vi "SW_Load_data_for_Analysis_from_TDMS.vi"(4 "Data samples to load":i64=-1, 6 "create index file? (T)":bool, 8 "error in (no error)":errorcluster, 9 "Progress bar reference":refnum<vi>, 10 "Cluster of paths input":T3, 11 "Data flow controls":T4) -> (0 "error out":errorcluster, 2 "Time to load, ms":u32, 3 "Loaded data":T1={"Absolute timestamp (DBL)"=[], "Relative timestamp (DBL)"=[], "Zones normalized allocation array"=[], "Coordinates and speed"=[], "Current zone and TTLs"=[], "Acquisition settings cluster out"={"Researcher name"="", "N segments MIDFIELD"=0, "N segments BORDER"=0, "Radius, mm CENTER"=0, "Radius, mm MIDFIELD"=0, "Starting angle MIDFIELD"=0, "Starting angle BORDER"=0, "Cage diameter, mm"=0, "Bridge swap"=FALSE, "Bridge V. offset"=0.0, "Twisted neck"=FALSE, "Offset H."=0.0, "Name prefix"="SavedTrack", "Stop at"=0.0, "\"Stop at\" enabled"=FALSE, "Settings loaded OK"=FALSE}, "Stimulus presets array"=[]} {"Acquisition settings cluster out"."Stop at" format="%<%H:%M:%S>t"}, 5 "Data loaded OK":bool, 7 "Settings loaded OK":bool)   [LabVIEW 2018, in "Tracker.lvlib"]
uses:
  Tracker.lvlib
panel:
  out "Author's name":string
  out "Stimulus presets array (loaded)":T2(array[cluster])
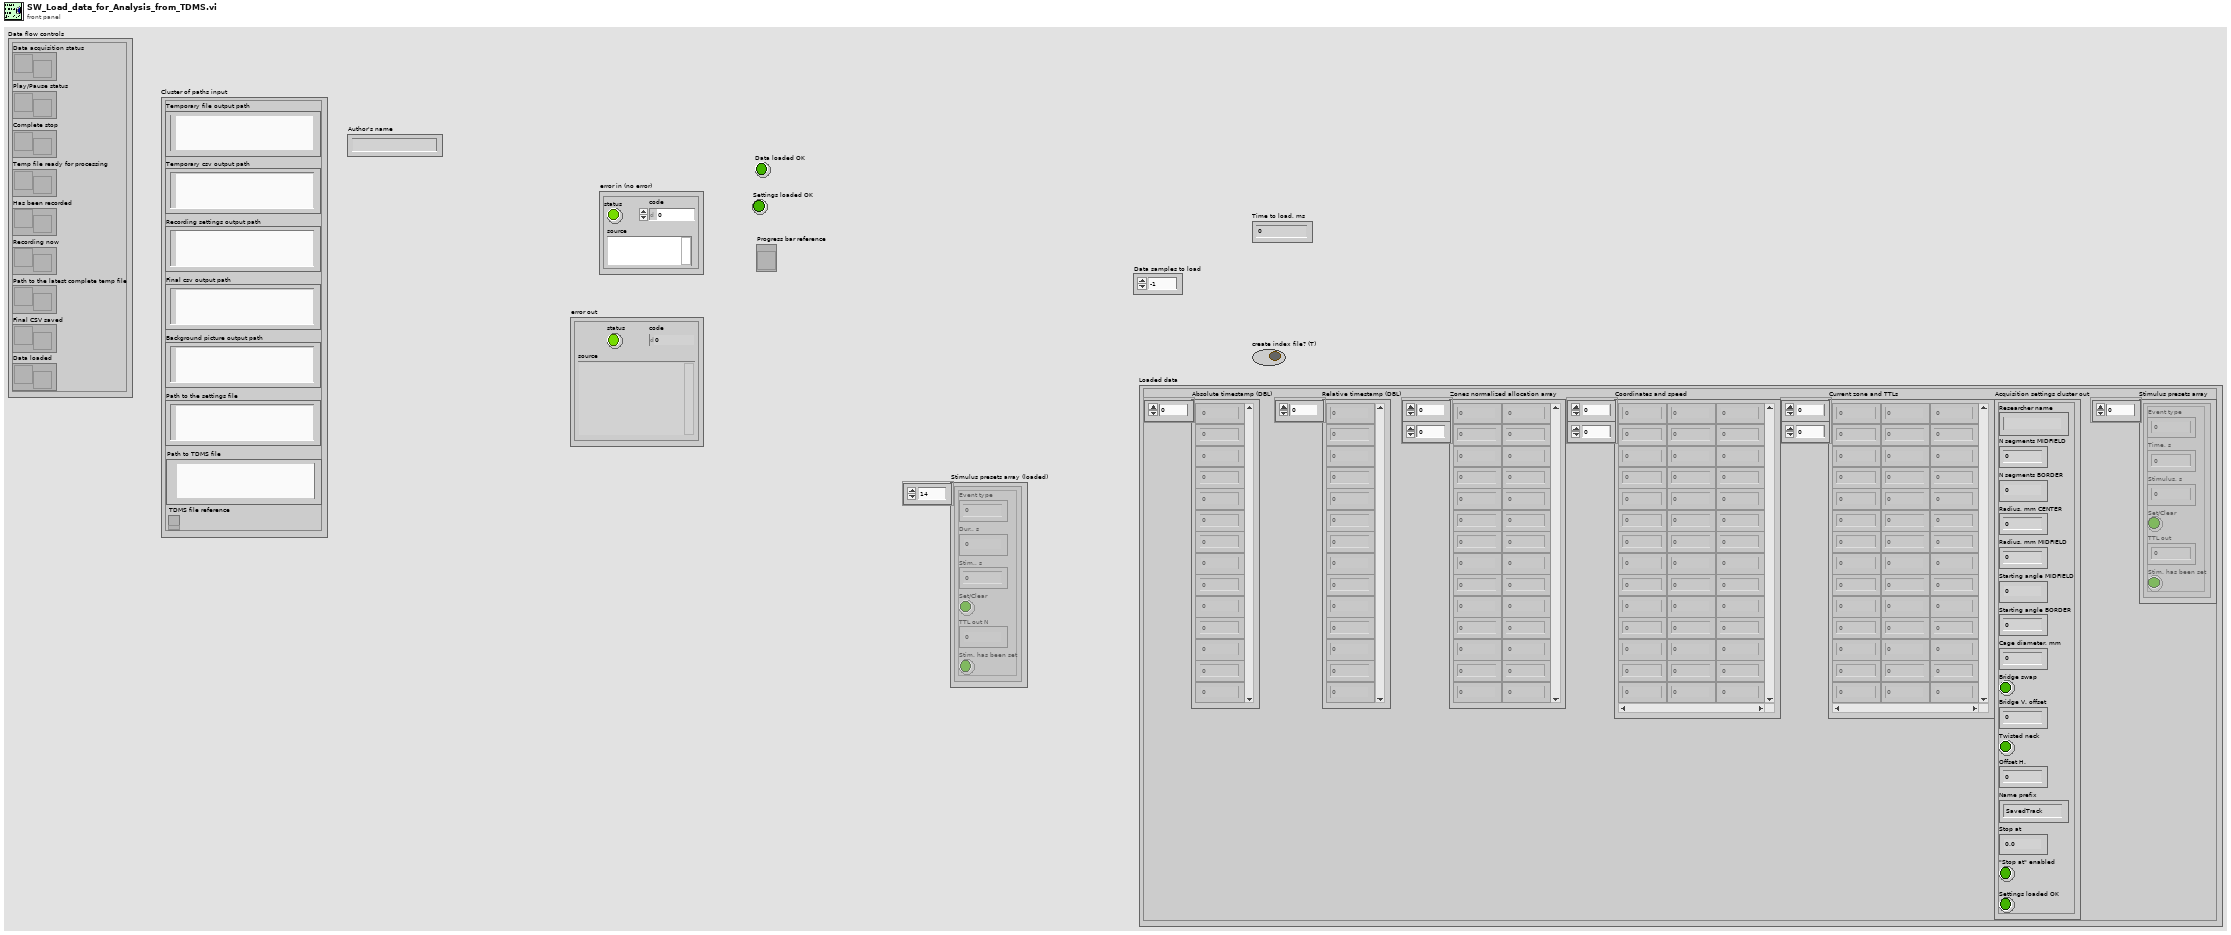
[diagram p1: front panel]
types:
  T1 = cluster{"Absolute timestamp (DBL)":dbl[], "Relative timestamp (DBL)":dbl[], "Zones normalized allocation array":dbl[][], "Coordinates and speed":dbl[][], "Current zone and TTLs":u8[][], "Acquisition settings cluster out":cluster{"Researcher name":string, "N segments MIDFIELD":u8, "N segments BORDER":u8, "Radius, mm CENTER":u16, "Radius, mm MIDFIELD":u16, "Starting angle MIDFIELD":i16, "Starting angle BORDER":i16, "Cage diameter, mm":u16, "Bridge swap":bool, "Bridge V. offset":sgl, "Twisted neck":bool, "Offset H.":sgl, "Name prefix":string, "Stop at":dbl, "\"Stop at\" enabled":bool, "Settings loaded OK":bool}, "Stimulus presets array":cluster{"Event type":u16, "Time, s":sgl, "Stimulus, s":sgl, "Set/Clear":bool, "TTL out":u16, "Stim. has been set":bool}[]}
  T2 = cluster{"Event type":u16, "Dur., s":sgl, "Stim., s":sgl, "Set/Clear":bool, "TTL out N":u16, "Stim. has been set":bool}[]
  T3 = cluster{"Temporary file output path":path, "Temporary csv output path":path, "Recording settings output path":path, "Final csv output path":path, "Background picture output path":path, "Path to the settings file":path, "Path to TDMS file":path, "TDMS file reference":refnum<k34>}
  T4 = cluster{"Data acquisition status":refnum<notifier>, "Play/Pause status":refnum<notifier>, "Complete stop":refnum<notifier>, "Temp file ready for processing":refnum<notifier>, "Has been recorded":refnum<notifier>, "Recording now":refnum<notifier>, "Path to the latest complete temp file":refnum<notifier>, "Final CSV saved":refnum<notifier>, "Data loaded":refnum<notifier>}
  T5 = cluster{"N segments BORDER":u8, "Starting angle BORDER":i16, "N segments MIDFIELD":u8, "Starting angle MIDFIELD":i16, "Radius, mm MIDFIELD":u16, "Amount of central segments":u8, "Radius, mm CENTER":u16, "Bridge swap":bool, "Bridge V. offset":sgl, "Twisted neck":bool, "Offset H.":sgl, "Zones configuration":string[], "IO parameters string":string, "Cage diameter, mm":u16, "Name prefix":string, "Stop at":dbl, "\"Stop at\" enabled":bool}
  T6 = enum16{"big-endian, network order", "native, host order", "little-endian"}
  T7 = enum16{"open", "open or create", "create or replace", "create", "open (read-only)"}
  T8 = cluster{"N segments BORDER":u8, "Starting angle BORDER":i16, "N segments MIDFIELD":u8, "Starting angle MIDFIELD":i16, "Radius, mm MIDFIELD":u16, "Amount of central segments":u8, "Radius, mm CENTER":u16, "Bridge offset":sgl, "Bridge swap":bool, "Zones configuration":string[], "IO parameters string":string, "Cage diameter, mm":u16}
  T9 = cluster{"Event type":u16, "Time, s":sgl, "Stimulus, s":sgl, "Set/Clear":bool, "TTL out":u16, "Stim. has been set":bool}
  T10 = cluster{string, "N segments MIDFIELD":u8, "N segments BORDER":u8, "Radius, mm CENTER":u16, "Radius, mm MIDFIELD":u16, "Starting angle MIDFIELD":i16, "Starting angle BORDER":i16, "Cage diameter, mm":u16, "Bridge swap":bool, "Bridge V. offset":sgl, "Twisted neck":bool, "Offset H.":sgl, "Name prefix":string, "Stop at":dbl, "\"Stop at\" enabled":bool, bool}
  T11 = cluster{dbl[], dbl[], "Zones normalized allocation array":dbl[][], dbl[][], u8[][], cluster{string, "N segments MIDFIELD":u8, "N segments BORDER":u8, "Radius, mm CENTER":u16, "Radius, mm MIDFIELD":u16, "Starting angle MIDFIELD":i16, "Starting angle BORDER":i16, "Cage diameter, mm":u16, "Bridge swap":bool, "Bridge V. offset":sgl, "Twisted neck":bool, "Offset H.":sgl, "Name prefix":string, "Stop at":dbl, "\"Stop at\" enabled":bool, bool}, cluster{"Event type":u16, "Time, s":sgl, "Stimulus, s":sgl, "Set/Clear":bool, "TTL out":u16, "Stim. has been set":bool}[]}
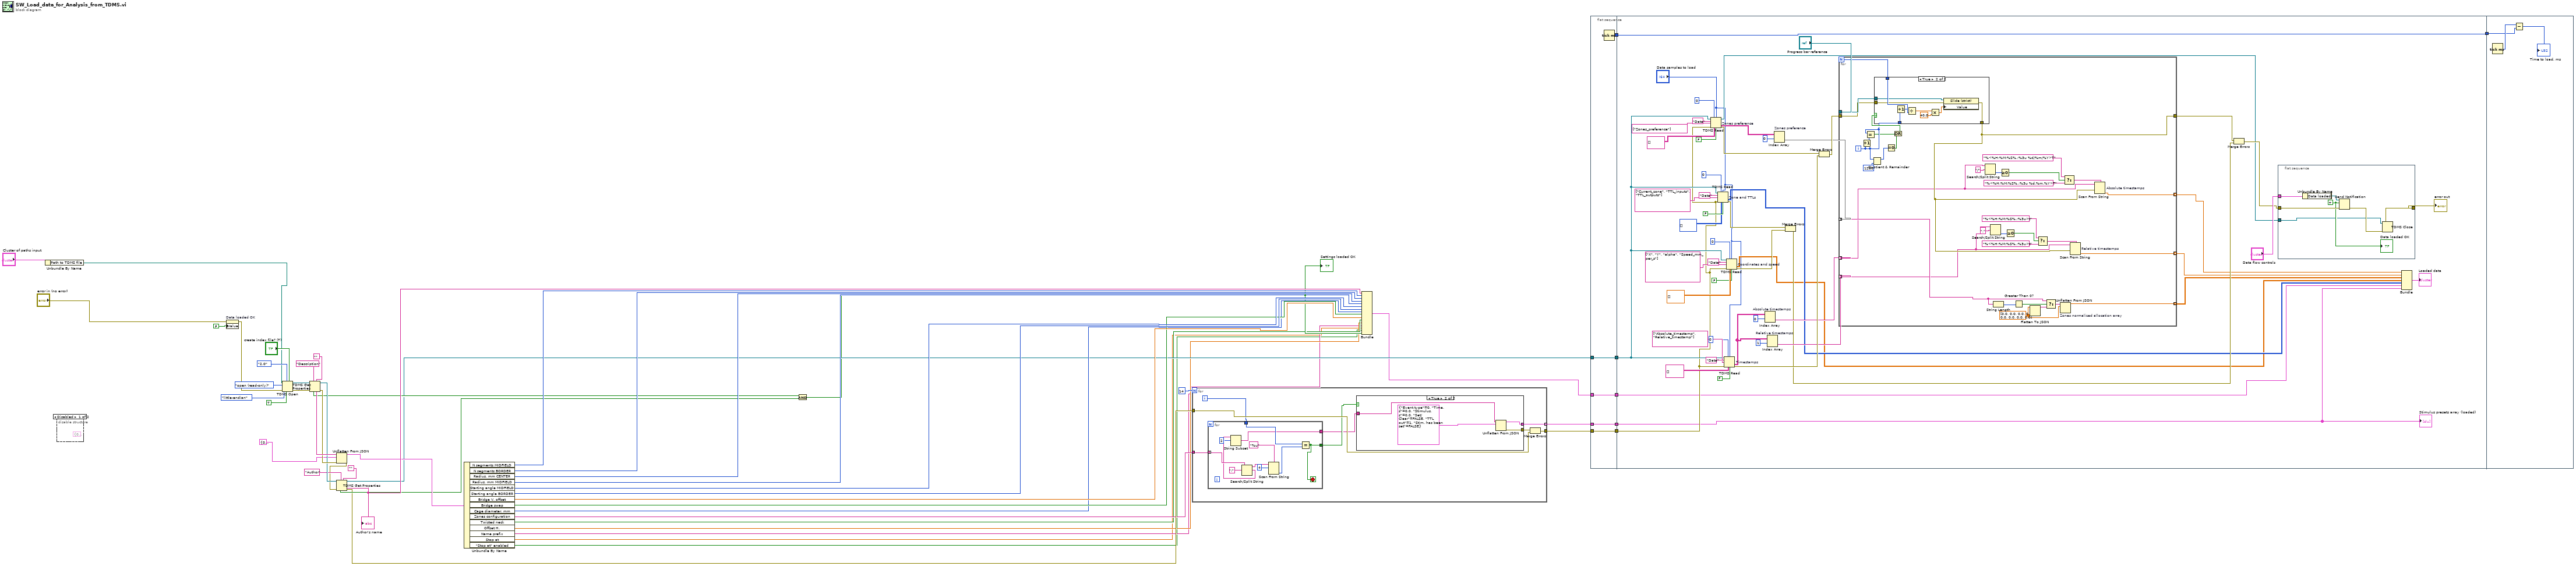
[diagram p0: block diagram]
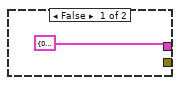
[diagram p4: hidden frame]
diagram:
  n1 = Unbundle By Name("Cluster of paths input") -> ("Path to TDMS file"=w9:path)
  n2 = disable-structure shown="Disabled" {
    frame Disabled {
      (unwired) T8 {"N segments BORDER"=0, "Starting angle BORDER"=0, "N segments MIDFIELD"=0, "Starting angle MIDFIELD"=0, "Radius, mm MIDFIELD"=0, "Amount of central segments"=0, "Radius, mm CENTER"=0, "Bridge offset"=0.0, "Bridge swap"=FALSE, "Zones configuration"=[], "IO parameters string"="[12,1,1,0,0,0]", "Cage diameter, mm"=180} ("Parameters")
    }
    frame Enabled {
    }
  }
  n3 = property on="Data loaded OK" class="Bool (strict)"(error in="error in (no error)", "Value"=FALSE ("Data loaded OK")) -> (error out=w17:errorcluster)  [unwired: 1 in, 1 out]
  n4 = TDMS Open(5:"create index file? (T)", 6:TRUE ("disable buffering? (T)"), 7:enum16{"1.0", "2.0"}."2.0" ("file format version (2.0)"), 8:w17, 9:T6."little-endian" ("byte order (2:little-endian)"), 10:T7."open (read-only)" ("operation (0:open)"), 11:w9) -> (0:w46:errorcluster, 3:w47:refnum<k34>)
  n5 = TDMS Get Properties(5:"", 7:"Description" ("property name"), 8:w46, 11:w47) -> (0:w42:errorcluster, 3:w41:refnum<k34>, 4:w43:string, 6:w26:bool)  [unwired: 2 in, 2 out]
  n6 = Unflatten From JSON(JSON string=w43, type and defaults=T5 {"N segments BORDER"=0, "Starting angle BORDER"=0, "N segments MIDFIELD"=0, "Starting angle MIDFIELD"=0, "Radius, mm MIDFIELD"=0, "Amount of central segments"=0, "Radius, mm CENTER"=0, "Bridge swap"=FALSE, "Bridge V. offset"=0.0, "Twisted neck"=FALSE, "Offset H."=0.0, "Zones configuration"=[], "IO parameters string"="[12,1,1,0,0,0]", "Cage diameter, mm"=180, "Name prefix"="SavedTrack", "Stop at"=0.0, "\"Stop at\" enabled"=FALSE} ("Parameters"), error in (no error)=w42) -> (value=w28:T5, error out=w38:errorcluster)  [unwired: 4 in]
  n7 = TDMS Get Properties(5:"", 7:"Author" ("property name"), 8:w38, 11:w41) -> (0:w24:errorcluster, 3:w21:refnum<k34>, 4:w37:string, 6:w25:bool)  [unwired: 2 in, 2 out]
  "Author's name" <- w37
  n8 = Unbundle By Name(w28) -> ("N segments MIDFIELD"=w36:u8, "N segments BORDER"=w35:u8, "Radius, mm CENTER"=w34:u16, "Radius, mm MIDFIELD"=w33:u16, "Starting angle MIDFIELD"=w32:i16, "Starting angle BORDER"=w31:i16, "Bridge V. offset"=w30:sgl, "Bridge swap"=w29:bool, "Cage diameter, mm"=w27:u16, "Zones configuration"=w23:string[], "Twisted neck"=w5:bool, "Offset H."=w4:sgl, "Name prefix"=w3:string, "Stop at"=w2:dbl, "\"Stop at\" enabled"=w1:bool)
  n9 = And(x=w26, y=w25) -> (x .and. y?=w6:bool)
  "Settings loaded OK" <- w6
  n10 = for {
    N: 14 -> [_]
    tunnel: w24 -> [w58]
    tunnel: [w60] -> w20
    tunnel: [w61] -> w19 mode=indexing
    tunnel: w23 -> [w56]
    i -> [w57]
    n11 = for {
      tunnel: w56 -> [w72] mode=indexing
      tunnel: w57 -> [w66]
      tunnel: [w65] -> w55
      tunnel: [w64] -> w54
      stop <- w65 stop-if-true
      n12 = Search/Split String(string=w72, search string/char (-)=":") -> (substring before match=w70:string, match + rest of string=w63:string)  [unwired: 1 in, 1 out]
      n13 = String Subset(string=w63, offset (0)=2) -> (substring=w64:string)  [unwired: 1 in]
      n14 = Scan From String(format string="%u", input string=w70, initial scan location=u32 4) -> (output 1=w67:u32)  [unwired: 2 in, 3 out]
      n15 = Equal?(x=w66, y=w67) -> (x = y?=w65:bool)
    }
    n16 = case shown="True" w55 {
      tunnel: w54 -> [_ w77]
      tunnel: [T9 {"Event type"=0, "Time, s"=0.0, "Stimulus, s"=0.0, "Set/Clear"=FALSE, "TTL out"=1, "Stim. has been set"=FALSE} ("Cluster of the stimuls settings") w76] -> w61
      tunnel: [_ w75] -> w59
      frame False {
      }
      frame True {
        n17 = Unflatten From JSON(JSON string=w77, type and defaults=T9 {"Event type"=0, "Time, s"=0.0, "Stimulus, s"=0.0, "Set/Clear"=FALSE, "TTL out"=1, "Stim. has been set"=FALSE} ("Cluster of the stimuls settings")) -> (value=w76:T9, error out=w75:errorcluster)  [unwired: 5 in]
      }
    }
    n18 = Merge Errors(w59, w58) -> (w60:errorcluster)
  }
  n19 = Bundle(w37, "N segments MIDFIELD"=w36, "N segments BORDER"=w35, "Radius, mm CENTER"=w34, "Radius, mm MIDFIELD"=w33, "Starting angle MIDFIELD"=w32, "Starting angle BORDER"=w31, "Cage diameter, mm"=w27, "Bridge swap"=w29, "Bridge V. offset"=w30, "Twisted neck"=w5, "Offset H."=w4, "Name prefix"=w3, "Stop at"=w2, "\"Stop at\" enabled"=w1, w6) -> (w8:T10)  [unwired: 1 in]
  n20 = flat-sequence {
    tunnel: w19 -> [w79]
    tunnel: w8 -> [w80]
    tunnel: w20 -> [w81]
    tunnel: w21 -> [w82]
    tunnel: [w82] -> w15
    tunnel: [w81] -> w14
    tunnel: [w80] -> w13
    tunnel: [w79] -> w12
    tunnel: [w78] -> w11
    tunnel: w15 -> [w117]
    tunnel: w14 -> [w116]
    tunnel: w13 -> [w83]
    tunnel: w12 -> [w95]
    tunnel: w11 -> [w84]
    tunnel: [w84] -> w10
    tunnel: w10 -> [w187]
    frame #0 {
      n21 = Tick Count (ms)() -> (millisecond timer value=w78:u32)
    }
    frame #1 {
      n22 = TDMS Read "Zones preference"(0:w117, 1:i64 0 ("offset (0)"), 2:"Data samples to load", 5:"Data" ("group name in"), 7:string[] ["Zones_preference"] ("Columns Names"), 11:w116, 12:string[][] [], 13:FALSE ("return channels in file order? (F)")) -> (4:w90:refnum<k34>, 10:w102:string[][], 15:w113:errorcluster)  [unwired: 3 out]
      n23 = TDMS Read "Zone and TTLs"(0:w117, 1:i64 0 ("offset (0)"), 2:"Data samples to load", 5:"Data" ("group name in"), 7:string[] ["Current_zone", "TTL_inputs", "TTL_outputs"] ("Columns Names"), 11:w116, 12:u8[][] [], 13:FALSE ("return channels in file order? (F)")) -> (10:w93:u8[][], 15:w111:errorcluster)  [unwired: 4 out]
      n24 = TDMS Read "Timestamps"(0:w117, 1:i64 0 ("offset (0)"), 2:"Data samples to load", 5:"Data" ("group name in"), 7:string[] ["Absolute_timestamp", "Relative_timestamp"] ("Columns Names"), 11:w116, 12:string[][] [], 13:FALSE ("return channels in file order? (F)")) -> (10:w106:string[][], 15:w112:errorcluster)  [unwired: 4 out]
      n25 = TDMS Read "Coordinates and speed"(0:w117, 1:i64 0 ("offset (0)"), 2:"Data samples to load", 5:"Data" ("group name in"), 7:string[] ["X", "Y", "alpha", "Speed_mm_per_s"] ("Columns Names"), 11:w116, 12:dbl[][] [], 13:FALSE ("return channels in file order? (F)")) -> (10:w92:dbl[][], 15:w100:errorcluster)  [unwired: 4 out]
      n26 = Index Array "Absolute timestamps"(array=w106, index (row)=0) -> (element=w105:string[])  [unwired: 1 in]
      n27 = Index Array "Relative timestamps"(array=w106, index (row)=1) -> (element=w104:string[])  [unwired: 1 in]
      n28 = Index Array "Zones preference"(array=w102, index (row)=0) -> (element=w101:string[])  [unwired: 1 in]
      n29 = Merge Errors(w111, w100) -> (w99:errorcluster)
      n30 = Merge Errors(w113, w112) -> (w114:errorcluster)
      n31 = for {
        N -> [w168]
        tunnel: w114 -> [w166]
        tunnel: [w153] -> w110
        tunnel: "Progress bar reference" -> [w167]
        tunnel: w105 -> [w145] mode=indexing
        tunnel: w104 -> [w143] mode=indexing
        tunnel: w101 -> [w147] mode=indexing
        tunnel: [w146] -> w96 mode=indexing
        tunnel: [w144] -> w98 mode=indexing
        tunnel: [w142] -> w97 mode=indexing
        i -> [w137]
        w148 = dbl[] [0.0, 0.0, 0.0, 0.0, 0.0, 0.0, 0.0, 0.0, 0.0] ("Zones normalized allocation array")
        n32 = Increment(x=w137) -> (x+1=w135:i32)
        n33 = Equal?(x=w137, y=w135) -> (x = y?=w136:bool)
        n34 = Quotient & Remainder(x=w137, y=1200) -> (x-y*floor(x/y)=w140:i32)  [unwired: 1 out]
        n35 = Equal To 0?(x=w140) -> (x = 0?=w139:bool)
        n36 = Or(x=w136, y=w139) -> (x .or. y?=w138:bool)
        n37 = case shown="True" w138 {
          tunnel: w137 -> [_ w178]
          tunnel: w168 -> [_ w177]
          tunnel: w167 -> [_ w176]
          tunnel: w166 -> [w169 w175]
          tunnel: [w169 w174] -> w153
          frame False {
          }
          frame True {
            n38 = Increment(x=w178) -> (x+1=w171:i32)
            n39 = Divide(x=w171, y=w177) -> (x/y=w173:dbl)
            n40 = Multiply(x=w173, y=40.0) -> (x*y=w170:dbl)
            n41 = property on="Property Node" class="Slide (strict)"(reference=w176, error in=w175, "Value"=w170) -> (error out=w174:errorcluster)  [unwired: 1 out]
          }
        }
        n42 = Search/Split String(string=w145, search string/char (-)="/") -> (offset of match=w161:i32)  [unwired: 1 in, 2 out]
        n43 = Search/Split String(string=w143, search string/char (-)=".") -> (offset of match=w157:i32)  [unwired: 1 in, 2 out]
        n44 = String Length(string=w147) -> (length=w152:i32)
        n45 = Greater Or Equal To 0?(x=w161) -> (x >= 0?=w160:bool)
        n46 = Greater Or Equal To 0?(x=w157) -> (x >= 0?=w154:bool)
        n47 = Greater Than 0?(x=w152) -> (x > 0?=w151:bool)
        n48 = Flatten To JSON(anything=w148) -> (JSON string=w149:string)  [unwired: 2 in, 1 out]
        n49 = Select(t="%<%H:%M:%S%.;%3u>t" ("format string"), s=w154, f="%<%H:%M:%S%,;%3u>t" ("format string")) -> (s? t:f=w159:string)
        n50 = Select(t=w147, s=w151, f=w149) -> (s? t:f=w150:string)
        n51 = Unflatten From JSON "Zones normalized allocation array"(JSON string=w150, type and defaults=w148) -> (value=w146:dbl[])  [unwired: 5 in, 1 out]
        n52 = Select(t="%<%H:%M:%S%.;%3u %d/%m/%Y>T" ("format string"), s=w160, f="%<%H:%M:%S%,;%3u %d.%m.%Y>T" ("format string")) -> (s? t:f=w163:string)
        n53 = Scan From String "Relative timestamps"(format string=w159, input string=w143, error in=w153) -> (output 1=w142:dbl)  [unwired: 2 in, 3 out]
        n54 = Scan From String "Absolute timestamps"(format string=w163, input string=w145, error in=w153) -> (output 1=w144:dbl)  [unwired: 2 in, 3 out]
      }
      n55 = Merge Errors(w110, w99) -> (w109:errorcluster)
      n56 = flat-sequence {
        tunnel: "Data flow controls" -> [w185]
        tunnel: [w181] -> w91
        tunnel: w109 -> [w184]
        tunnel: w90 -> [w180]
        frame #0 {
          w183 = TRUE ("notification")
          n57 = Unbundle By Name(w185) -> ("Data loaded"=w179:refnum<notifier>)
          n58 = Send Notification(notification=w183, notifier=w179, error in (no error)=w184) -> (error out=w182:errorcluster)  [unwired: 1 out]
          n59 = TDMS Close(8:w182, 11:w180) -> (0:w181:errorcluster)  [unwired: 1 out]
          "Data loaded OK" <- w183
        }
      }
      n60 = Bundle(w98, w97, "Zones normalized allocation array"=w96, w92, w93, w83, w95) -> (→"Loaded data":T11)  [unwired: 1 in]
      "error out" <- w91
      "Stimulus presets array (loaded)" <- w95
    }
    frame #2 {
      n61 = Tick Count (ms)() -> (millisecond timer value=w188:u32)
      n62 = Subtract(x=w188, y=w187) -> (x-y=→"Time to load, ms":u32)
    }
  }
